vi "configureAcquisition.vi"(6 "imagePaths":path[](array[path]), 7 "saveImages?":bool, 8 "error in (no error)":errorcluster, 9 "number of Images":i32, 10 "CamaraSettings":refnum<class "CamaraSettings.lvclass">, 11 "NetworkProEM in":refnum<class "Network_ProEm_WinX32.lvclass">) -> (0 "error out":errorcluster, 3 "NetworkProEM out":refnum<class "Network_ProEm_WinX32.lvclass">)   [LabVIEW 2009, in "Hardware.lvlib" / "HWControllers.lvlib" / "Network_ProEm_WinX32.lvclass"]
uses:
  Network_ProEm_WinX32.lvclass
  Tools/CameraSettings/CamaraSettings.lvclass
  Channels/Camera/Camera/Camera.lvclass
  NetworkCamera.lvclass
panel:
  out "ImagesTaken":i32
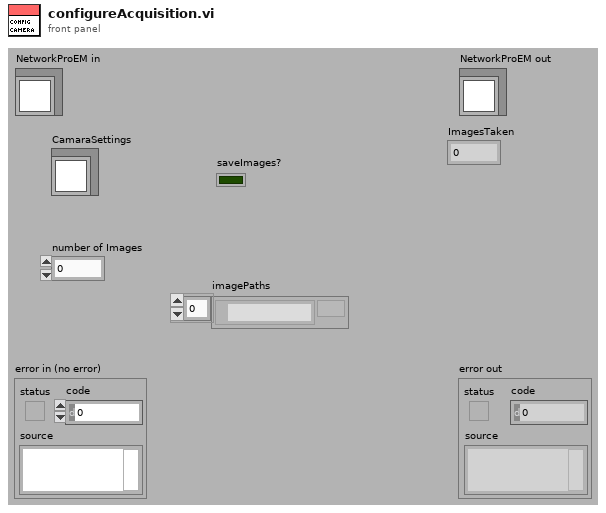
[diagram p1: front panel]
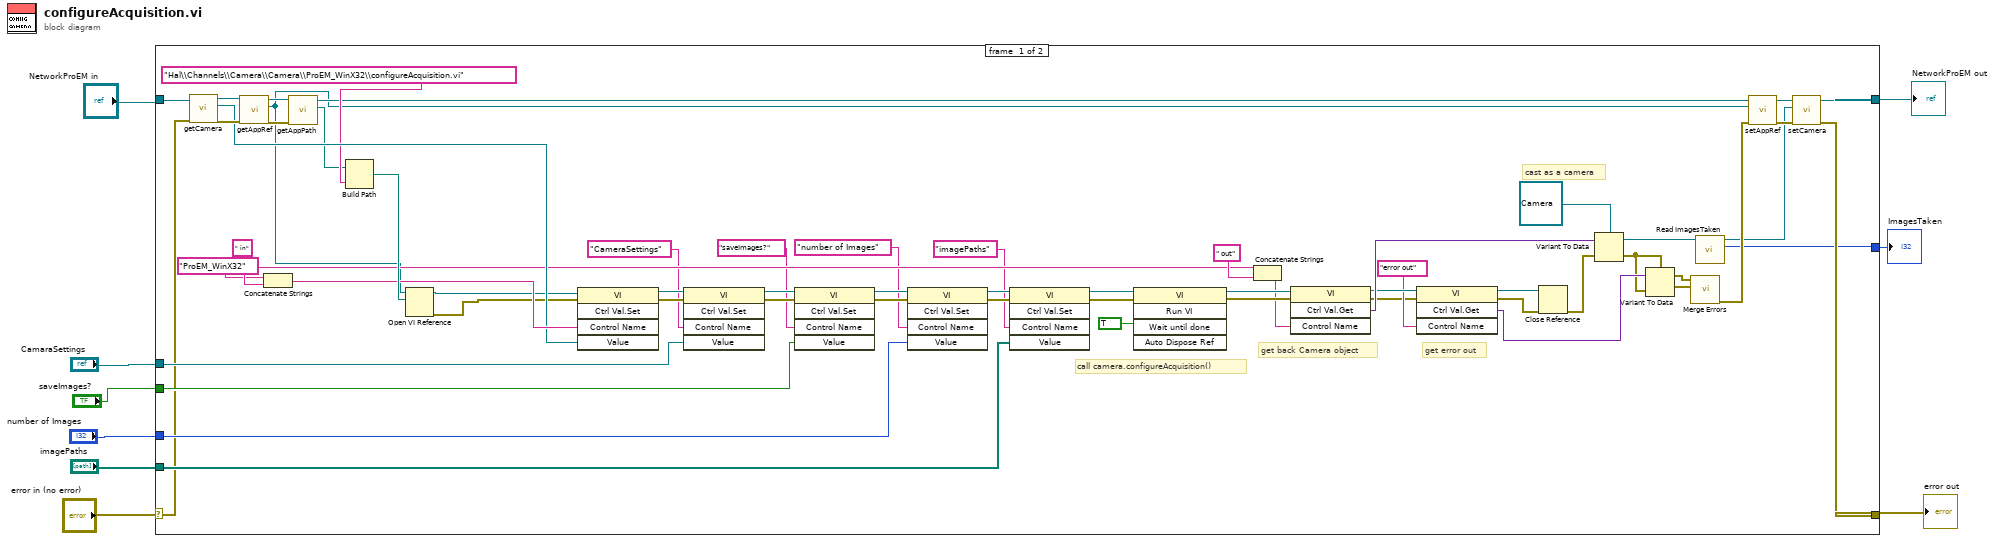
[diagram p0: block diagram]
diagram:
  n1 = case shown="No Error" "error in (no error)" {
    selector: "error in (no error)" -> [w18 w71]
    tunnel: [w45 w71] -> w7
    tunnel: [w47 w70] -> w8
    tunnel: "NetworkProEM in" -> [w53 w70]
    tunnel: "CamaraSettings" -> [w36 _]
    tunnel: "saveImages?" -> [w34 _]
    tunnel: "number of Images" -> [w33 _]
    tunnel: "imagePaths" -> [w28 _]
    tunnel: [w10 _] -> w1
    frame #0 {
      w50 = "ProEM_WinX32" ("Control name")
      # "get error out"
      # "get back Camera object"
      # "call camera.configureAcquisition()"
      # "cast as a camera"
      n2 = call "getCamera.vi"("error in (no error)"=w18, "NetworkCamera in"=w53) -> ("error out"=w56:errorcluster, "Camera"=w52:refnum<class "Camera.lvclass">, "NetworkCamera out"=w57:refnum<class "Network_ProEm_WinX32.lvclass">)  [unwired: 7 in]
      n3 = call "getAppRef.vi"("error in (no error)"=w56, "NetworkCamera in"=w57) -> ("error out"=w54:errorcluster, "appRef"=w17:refnum<vi>, "NetworkCamera out"=w55:refnum<class "Network_ProEm_WinX32.lvclass">)  [unwired: 7 in]
      n4 = Concatenate Strings(w50, " in") -> (w60:string)
      n5 = call "getAppPath.vi"("error in (no error)"=w54, "NetworkCamera in"=w55) -> ("appPath"=w16:path, "NetworkCamera out"=w49:refnum<class "Network_ProEm_WinX32.lvclass">)  [unwired: 7 in, 1 out]
      n6 = Build Path(base path=w16, name or relative path="Hal\\Channels\\Camera\\Camera\\ProEM_WinX32\\configureAcquisition.vi" ("viPath")) -> (appended path=w69:path)
      n7 = Open VI Reference(application reference (local)=w17, vi path=w69) -> (vi reference=w14:refnum<vi>, error out=w13:errorcluster)  [unwired: 4 in]
      n8 = invoke class="VI" method="Ctrl Val.Set"(reference=w14, error in=w13, "Control Name"=w60, "Value"=w52) -> (reference out=w44:refnum<vi>, error out=w40:errorcluster)  [unwired: 1 in, 3 out]
      n9 = invoke class="VI" method="Ctrl Val.Set"(reference=w44, error in=w40, "Control Name"="CameraSettings", "Value"=w36) -> (reference out=w43:refnum<vi>, error out=w39:errorcluster)  [unwired: 1 in, 3 out]
      n10 = invoke class="VI" method="Ctrl Val.Set"(reference=w43, error in=w39, "Control Name"="saveImages?", "Value"=w34) -> (reference out=w42:refnum<vi>, error out=w38:errorcluster)  [unwired: 1 in, 3 out]
      n11 = invoke class="VI" method="Ctrl Val.Set"(reference=w42, error in=w38, "Control Name"="number of Images", "Value"=w33) -> (reference out=w41:refnum<vi>, error out=w30:errorcluster)  [unwired: 1 in, 3 out]
      n12 = invoke class="VI" method="Ctrl Val.Set"(reference=w41, error in=w30, "Control Name"="imagePaths", "Value"=w28) -> (reference out=w31:refnum<vi>, error out=w27:errorcluster)  [unwired: 1 in, 3 out]
      n13 = invoke class="VI" method="Run VI"(reference=w31, error in=w27, "Wait until done"=TRUE) -> (reference out=w67:refnum<vi>, error out=w66:errorcluster)  [unwired: 2 in, 3 out]
      n14 = Concatenate Strings(w50, " out") -> (w58:string)
      n15 = invoke class="VI" method="Ctrl Val.Get"(reference=w67, error in=w66, "Control Name"=w58) -> (reference out=w63:refnum<vi>, error out=w24:errorcluster, "Get Control Value Variant"=w64:variant)  [unwired: 1 in, 1 out]
      n16 = invoke class="VI" method="Ctrl Val.Get"(reference=w63, error in=w24, "Control Name"="error out") -> (reference out=w26:refnum<vi>, error out=w15:errorcluster, "Get Control Value Variant"=w23:variant)  [unwired: 1 in, 1 out]
      n17 = Close Reference(reference=w26, error in (no error)=w15) -> (error out=w62:errorcluster)
      n18 = Variant To Data(error in=w62, Variant=w64, type=refnum<class "Camera.lvclass"> refnum ("Camera out")) -> (error out=w22:errorcluster, data=w12:refnum<class "Camera.lvclass">)
      n19 = Variant To Data(error in=w22, Variant=w23, type=w22) -> (error out=w20:errorcluster, data=w21:errorcluster)
      n20 = call <vilib>:"Merge Errors.vi"("error in 2 (no error)"=w20, "error in 1 (no error)"=w21) -> ("error out"=w19:errorcluster)  [unwired: 5 in]
      n21 = call "Read ImagesTaken.vi"("Camera in"=w12) -> ("ImagesTaken"=w10:i32, "Camera out"=w11:refnum<class "Camera.lvclass">)  [unwired: 8 in, 1 out]
      n22 = call "setAppRef.vi"("error in (no error)"=w19, "appRef"=w17, "NetworkCamera in"=w49) -> ("error out"=w46:errorcluster, "NetworkCamera out"=w48:refnum<class "Network_ProEm_WinX32.lvclass">)  [unwired: 7 in]
      n23 = call "setCamera.vi"("error in (no error)"=w46, "Camera"=w11, "NetworkCamera in"=w48) -> ("error out"=w45:errorcluster, "NetworkCamera out"=w47:refnum<class "Network_ProEm_WinX32.lvclass">)  [unwired: 7 in]
    }
    frame #1 {
    }
  }
  "error out" <- w7
  "NetworkProEM out" <- w8
  "ImagesTaken" <- w1
